vi "StringFactory.vi"(8 "error in":errorcluster, 11 "reference":refnum<vi>) -> (0 "error out":errorcluster, 3 "String out":refnum<class "String.lvclass">)   [LabVIEW 2014, in "Raspberry Pi Compatible Compiler for LabVIEW.lvlib" / "String.lvclass"]
uses:
  String.lvclass
  Combobox/Combobox.lvclass
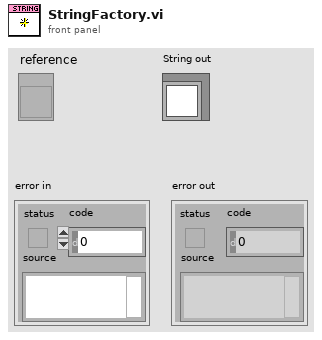
[diagram p1: front panel]
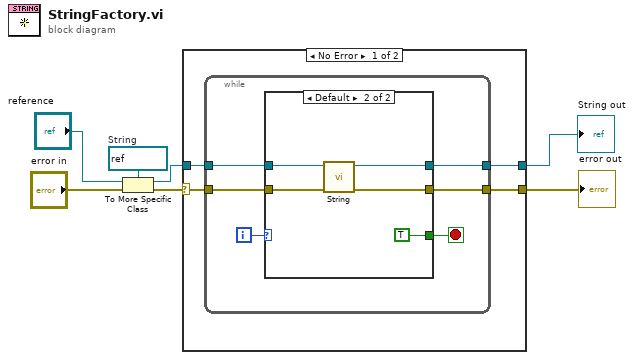
[diagram p0: block diagram]
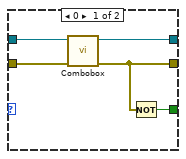
[diagram p2: hidden frame]
diagram:
  w7 = refnum<vi> refnum  # String
  n1 = To More Specific Class(target class=w7, reference="reference", error in="error in") -> (specific class reference=w3:refnum<vi>, error out=w4:errorcluster)
  n2 = case shown="No Error" w4 {
    selector: w4 -> [w11 w28]
    tunnel: [w9 _] -> w2
    tunnel: [w8 w28] -> w1
    tunnel: w3 -> [w10 _]
    frame No Error {
      n3 = while {
        tunnel: w11 -> [w16]
        tunnel: [w15] -> w8
        tunnel: [w14] -> w9
        tunnel: w10 -> [w12]
        i -> [w17]
        stop <- w13 stop-if-true
        n4 = case shown="Default" w17 {
          tunnel: w16 -> [w22 w25]
          tunnel: [w19 w23] -> w15
          tunnel: [w21 w24] -> w14
          tunnel: [w20 TRUE] -> w13
          tunnel: w12 -> [w18 w26]
          frame 0 {
            n5 = call "Combobox.vi"("error in"=w22, "GObj Refnum"=w18) -> ("error out"=w19:errorcluster, "Combobox out"=w21:refnum<class "Combobox.lvclass">)  [unwired: 8 in]
            n6 = Not(x=w19) -> (.not. x?=w20:bool)
          }
          frame Default {
            n7 = call "String.vi"("error in"=w25, "GObj Refnum"=w26) -> ("error out"=w23:errorcluster, "String out"=w24:refnum<class "String.lvclass">)  [unwired: 8 in]
          }
        }
      }
    }
    frame Error {
    }
  }
  "error out" <- w1
  "String out" <- w2
